vi "DAC Configure FP View.vi"(8 "error in":errorcluster, 11 "DAC FTCU in":refnum<class "DAC FTCU.lvclass">) -> (0 "error out":errorcluster, 3 "DAC FTCU out":refnum<class "DAC FTCU.lvclass">)   [LabVIEW 2019, in "DAC.lvlib" / "DAC FTCU.lvclass"]
uses:
  DAC FTCU.lvclass
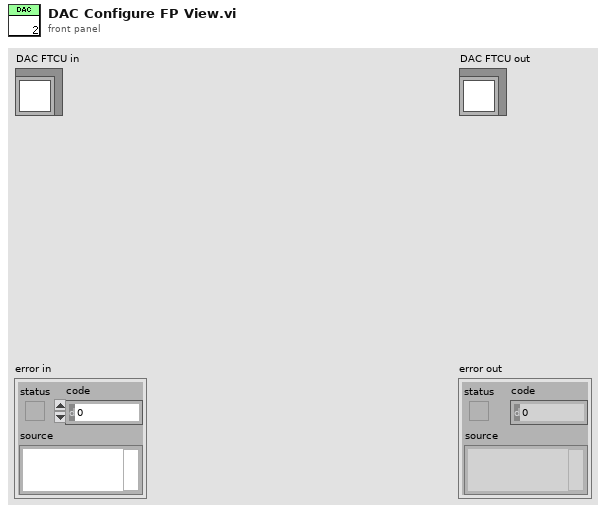
[diagram p1: front panel]
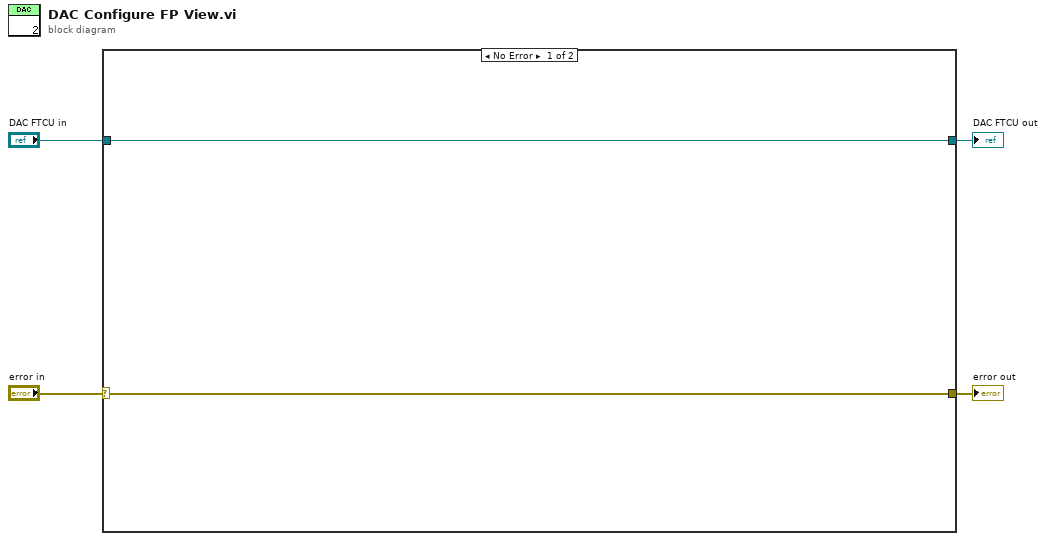
[diagram p0: block diagram]
diagram:
  n1 = case shown="No Error" "error in" {
    selector: "error in" -> [w5 w8]
    tunnel: [w5 w8] -> w1
    tunnel: [w6 w7] -> w2
    tunnel: "DAC FTCU in" -> [w6 w7]
    frame No Error {
    }
    frame Error {
    }
  }
  "error out" <- w1
  "DAC FTCU out" <- w2
